vi "Globals.vi"() -> ()   [LabVIEW 2019]
uses:
  TypeDef/Cluster NI.ctl
  SubVI/cDAQ_PLC Folder/controls/StatoAO_cdaq.ctl
  SubVI/cDAQ_PLC Folder/controls/statoDO_Cdaq.ctl
panel:
  out "LOG DATI?":bool
  out "new data?":bool
  out "SETUP":string[][](array[string])
  out "ERRORI MEDIE":dbl[](array[numeric])
  out "SLIDE":u8
  out "NPSH3":string
  in  "DATI TARGA":string[][](array[string])
  out "STOP AQ":bool
  out "Dati Costruttivi":string[](array[string])
  out "Dati Targa":string[](array[string])
  out "TIME offset [s]":dbl
  out "TIME [s]":dbl
  out "NM?":bool
  out "MONITOR 2":u8
  out "LINEA Q":i32
  out "V SIGMA":dbl
  out "PAUSA CICLO":bool
  out "NPSH?":bool
  out "NI READ":T1 {"AI (4-20mA)"."AI 15" format="%#_6f"; "AI (4-20mA)"."AI 14" format="%#_6f"; "AI (4-20mA)"."AI 13" format="%#_6f"; "AI (4-20mA)"."AI 11" format="%#_6f"; "AI (4-20mA)"."AI 10" format="%#_6f"; "AI (4-20mA)"."AI 9" format="%#_6f"; "AI (4-20mA)"."AI 4" format="%#_6f"; "AI (4-20mA)"."AI 12" format="%#_6f"; "AI (4-20mA)"."AI 0" format="%#_6f"; "AI (4-20mA)"."AI 1" format="%#_6f"; "AI (4-20mA)"."AI 2" format="%#_6f"; "AI (4-20mA)"."AI 3" format="%#_6f"; "AI (4-20mA)"."AI 5" format="%#_6f"; "AI (4-20mA)"."AI 6" format="%#_6f"; "AI (4-20mA)"."AI 7" format="%#_6f"; "AI (4-20mA)"."AI 8" format="%#_6f"; "AI (0-10V)"."AI 31" format="%#_6f"; "AI (0-10V)"."AI 30" format="%#_6f"; "AI (0-10V)"."AI 29" format="%#_6f"; "AI (0-10V)"."AI 28" format="%#_6f"; "AI (0-10V)"."AI 27" format="%#_6f"; "AI (0-10V)"."AI 26" format="%#_6f"; "AI (0-10V)"."AI 25" format="%#_6f"; "AI (0-10V)"."AI 24" format="%#_6f"; "AI (0-10V)"."AI 23" format="%#_6f"; "AI (0-10V)"."AI 22" format="%#_6f"; "AI (0-10V)"."AI 21" format="%#_6f"; "AI (0-10V)"."AI 20" format="%#_6f"; "AI (0-10V)"."AI 19" format="%#_6f"; "AI (0-10V)"."AI 18" format="%#_6f"; "AI (0-10V)"."AI 17" format="%#_6f"; "AI (0-10V)"."AI 16" format="%#_6f"; "AI (0-10V)"."AI 15" format="%#_6f"; "AI (0-10V)"."AI 14" format="%#_6f"; "AI (0-10V)"."AI 13" format="%#_6f"; "AI (0-10V)"."AI 11" format="%#_6f"; "AI (0-10V)"."AI 10" format="%#_6f"; "AI (0-10V)"."AI 9" format="%#_6f"; "AI (0-10V)"."AI 4" format="%#_6f"; "AI (0-10V)"."AI 12" format="%#_6f"; "AI (0-10V)"."AI 0" format="%#_6f"; "AI (0-10V)"."AI 1" format="%#_6f"; "AI (0-10V)"."AI 2" format="%#_6f"; "AI (0-10V)"."AI 3" format="%#_6f"; "AI (0-10V)"."AI 5" format="%#_6f"; "AI (0-10V)"."AI 6" format="%#_6f"; "AI (0-10V)"."AI 7" format="%#_6f"; "AI (0-10V)"."AI 8" format="%#_6f"}
  out "STOP":bool
  out "PASSO SALVATO":u8
  out "STOP CICLO":bool
  out "MONITOR 1":u8
  out "MANUALE?":bool
  out "Simulazione":bool
  in  "ESITO TEST":enum16{"IN CORSO", "OK", "KO"}(ring)
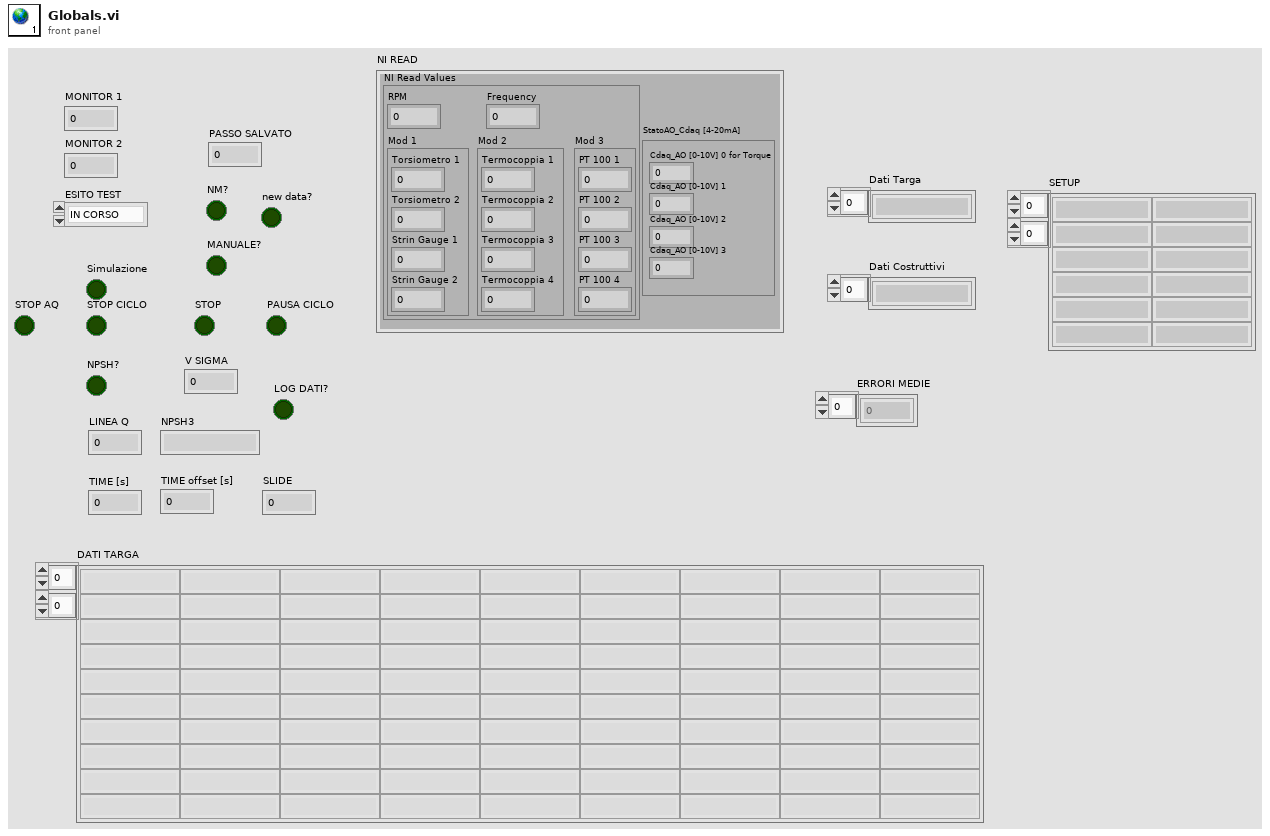
[diagram p1: front panel]
types:
  T1 = typedef "Cluster NI.ctl" = cluster{"AI (0-10V)":cluster{"AI 0":dbl, "AI 1":dbl, "AI 2":dbl, "AI 3":dbl, "AI 4":dbl, "AI 5":dbl, "AI 6":dbl, "AI 7":dbl, "AI 8":dbl, "AI 9":dbl, "AI 10":dbl, "AI 11":dbl, "AI 12":dbl, "AI 13":dbl, "AI 14":dbl, "AI 15":dbl, "AI 16":dbl, "AI 17":dbl, "AI 18":dbl, "AI 19":dbl, "AI 20":dbl, "AI 21":dbl, "AI 22":dbl, "AI 23":dbl, "AI 24":dbl, "AI 25":dbl, "AI 26":dbl, "AI 27":dbl, "AI 28":dbl, "AI 29":dbl, "AI 30":dbl, "AI 31":dbl}, "StatoAO_Cdaq[0-10V]":cluster{"AO 1":dbl, "AO 2":dbl, "AO 3":dbl, "AO 4":dbl}, "Contatori [rpm]":cluster{"RPM 1":dbl, "RPM 2":dbl}, "StatoAO_Cdaq [4-20mA]":T2, "StatoDO_Cdaq":T3, "DI":cluster{"Scorta 0":bool, "Scorta 1":bool, "Scorta 2":bool, "Scorta 3":bool, "Scorta 4":bool, "Scorta 5":bool, "Scorta 6":bool, "Scorta 7":bool, "Scorta 8":bool, "Scorta 9":bool, "Scorta 10":bool, "Scorta 11":bool, "Scorta 12":bool, "Scorta 13":bool, "Scorta 14":bool, "Scorta 15":bool, "Scorta 16":bool, "Scorta 17":bool, "Scorta 18":bool, "Scorta 19":bool, "Scorta 20":bool, "Scorta 21":bool, "Scorta 22":bool, "Scorta 23":bool, "Scorta 24":bool, "Scorta 25":bool, "Scorta 26":bool, "Scorta 27":bool, "Scorta 28":bool, "Scorta 29":bool, "Scorta 30":bool, "Scorta 31":bool}, "AI (4-20mA)":cluster{"AI 0":dbl, "AI 1":dbl, "AI 2":dbl, "AI 3":dbl, "AI 4":dbl, "AI 5":dbl, "AI 6":dbl, "AI 7":dbl, "AI 8":dbl, "AI 9":dbl, "AI 10":dbl, "AI 11":dbl, "AI 12":dbl, "AI 13":dbl, "AI 14":dbl, "AI 15":dbl}, "TC [°C]":cluster{"tc 1":dbl, "tc 2":dbl, "tc 3":dbl, "tc 4":dbl}, "NI Read Values":cluster{"RPM":dbl, "Frequency":dbl, "Mod 1":cluster{"Torsiometro 1":dbl, "Torsiometro 2":dbl, "Strin Gauge 1":dbl, "Strin Gauge 2":dbl}, "Mod 2":cluster{"Termocoppia 1":dbl, "Termocoppia 2":dbl, "Termocoppia 3":dbl, "Termocoppia 4":dbl}, "Mod 3":cluster{"PT 100 1":dbl, "PT 100 2":dbl, "PT 100 3":dbl, "PT 100 4":dbl}}}
  T2 = typedef "StatoAO_cdaq.ctl" = cluster{"Cdaq_AO [0-10V] 0 for Torque":dbl, "Cdaq_AO [0-10V] 1":dbl, "Cdaq_AO [0-10V] 2":dbl, "Cdaq_AO [0-10V] 3":dbl}
  T3 = typedef "statoDO_Cdaq.ctl" = cluster{"Scorta 0":bool, "Scorta 1":bool, "Scorta 2":bool, "Scorta 3":bool, "Scorta 4":bool, "Scorta 5":bool, "Scorta 6":bool, "Scorta 7":bool, "Scorta 8":bool, "Scorta 9":bool, "Scorta 10":bool, "Scorta 11":bool, "Scorta 12":bool, "Scorta 13":bool, "Scorta 14":bool, "Scorta 15":bool, "Scorta 16":bool, "Scorta 17":bool, "Scorta 18":bool, "Scorta 19":bool, "Scorta 20":bool, "Scorta 21":bool, "Scorta 22":bool, "Scorta 23":bool, "Scorta 24":bool, "Scorta 25":bool, "Scorta 26":bool, "Scorta 27":bool, "Scorta 28":bool, "Scorta 29":bool, "Scorta 30":bool, "Scorta 31":bool}
diagram:
